vi "GFITS_ResyncQueue.vi"(6 "maxtries":i32=5, 7 "nd queue":bool, 9 "ID in":string, 10 "var name":string, 11 "RefNum in":T1) -> (0 "error out":errorcluster, 1 "str datatype":string, 2 "value out":string[][](array[string]), 3 "sync ok":bool)   [LabVIEW 2016]
uses:
  DBSHAND/private/vis/DatabaseHand_RefNum.ctl
  DBSHAND/private/vis/DatabaseHand_Element_Get(2DArr).vi
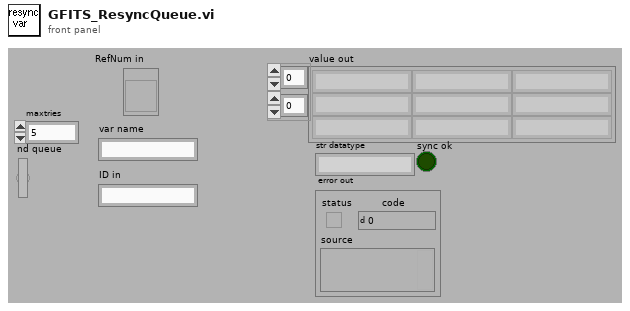
[diagram p1: front panel]
types:
  T1 = typedef "DatabaseHand_RefNum.ctl" = refnum<vi>
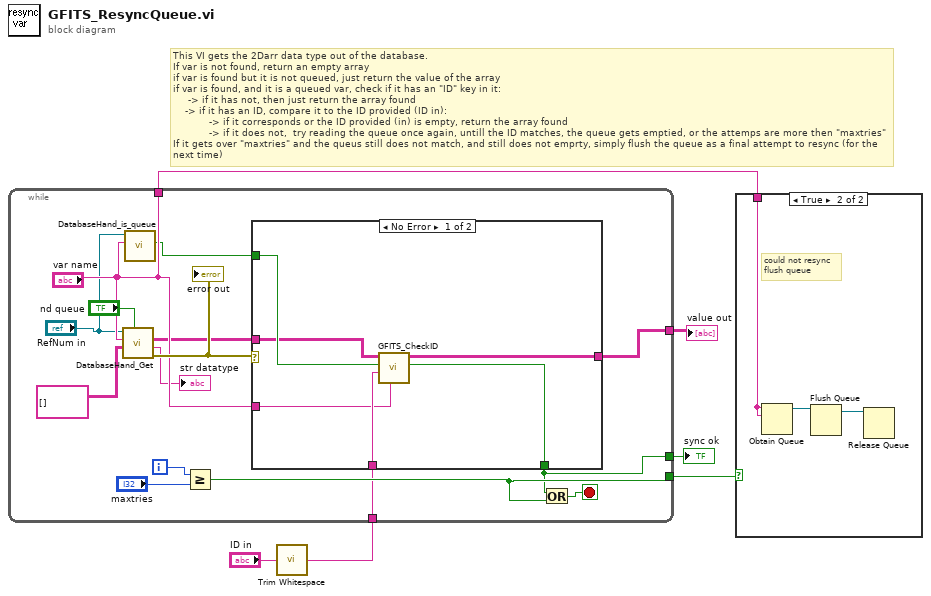
[diagram p0: block diagram]
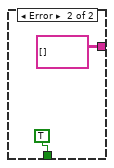
[diagram p3: hidden frame]
diagram:
  # "This VI gets the 2Darr data type out of the database.\nIf var is not found, return an empty array\nif var is found but it is not queued, just return the value of the array\nif var is found, and it is a queued var, check if it has an \"ID\" key in it:\n     -> if it has not, then just return the array found\n    -> if it has an ID, compare it to the ID provided (ID in):\n            -> if it corresponds or the ID provided (in) is empty, return the array found\n            -> if it does not,  try reading the queue once again, untill the ID matches, the queue gets emptied, or the attemps are more then \"maxtries\"\nIf it gets over \"maxtries\" and the queus still does not match, and still does not emprty, simply flush the queue as a final attempt to resync (for the next time)"
  n1 = call <vilib>:"Trim Whitespace.vi"("string"="ID in") -> ("trimmed string"=w2:string)  [unwired: 1 in]
  n2 = while {
    tunnel: [w21] -> w5
    tunnel: [w17] -> w6
    tunnel: ["var name"] -> w4
    tunnel: w2 -> [w16]
    tunnel: [w8] -> w1
    i -> [w19]
    stop <- w20 stop-if-true
    n3 = call-poly "DatabaseHand_Get.vi"("nd queue"="nd queue", "default value"=string[][] [], "name"="var name", "Database RefNum in"="RefNum in") -> ("error out"=w15:errorcluster, "type"=→"str datatype":string, "value"=w10:string[][])  [unwired: 1 in, 4 out]
    "error out" <- w15
    n4 = call "DatabaseHand_is_queue.vi"("name"="var name", "Database RefNum in"="RefNum in") -> ("queue?"=w12:bool)  [unwired: 1 in, 8 out]
    n5 = Greater Or Equal?(x=w19, y="maxtries") -> (x >= y?=w17:bool)
    n6 = case shown="No Error" w15 {
      tunnel: [w27 TRUE] -> w8
      tunnel: w12 -> [w26 _]
      tunnel: [w25 string[][] [] ("value out")] -> w21
      tunnel: w16 -> [w24 _]
      tunnel: "var name" -> [w23 _]
      tunnel: w10 -> [w22 _]
      frame No Error {
        n7 = call "GFITS_CheckID.vi"("array name"=w23, "expid"=w24, "queue?"=w26, "value"=w22) -> ("OK"=w27:bool, "value out"=w25:string[][])  [unwired: 6 out]
      }
      frame Error {
      }
    }
    n8 = Or(x=w8, y=w17) -> (x .or. y?=w20:bool)
  }
  "value out" <- w5
  "sync ok" <- w1
  n9 = case shown="True" w6 {
    tunnel: w4 -> [_ w30]
    frame False {
    }
    frame True {
      # "could not resync\nflush queue"
      n10 = Obtain Queue(name (unnamed)=w30, element data type=w30) -> (queue out=w32:refnum<queue>)  [unwired: 3 in, 2 out]
      n11 = Flush Queue(queue=w32) -> (queue out=w31:refnum<queue>)  [unwired: 1 in, 2 out]
      n12 = Release Queue(queue=w31) -> ()  [unwired: 1 in, 4 out]
    }
  }
